vi "读取数据.vi"(8 "error in (no error)":errorcluster, 10 "Slave ID":u8=1, 11 "MB session in":refnum<class "MB_Master.lvclass">) -> (0 "error out":errorcluster, 1 "Registers":u16[](array[numeric]), 2 "读取值":T1 {"累积流量单位" items=["L", "M3", "T", "USG"]; "瞬时流量单位" items=["L/S", "L/M", "L/H", "M3/S", "M3/M", "M3/H", "T/S", "T/M", "T/H", "GPS", "GPM", "GPH"]}, 3 "MB session out":refnum<class "MB_Master.lvclass">)   [LabVIEW 2016, in "MGG-KL-QC流量计.lvlib"]
uses:
  <vilib>/Plasmionique/MB Master/MB_Master/MB_Master.lvclass
  <vilib>/Plasmionique/MB Master/MB Master.lvlib
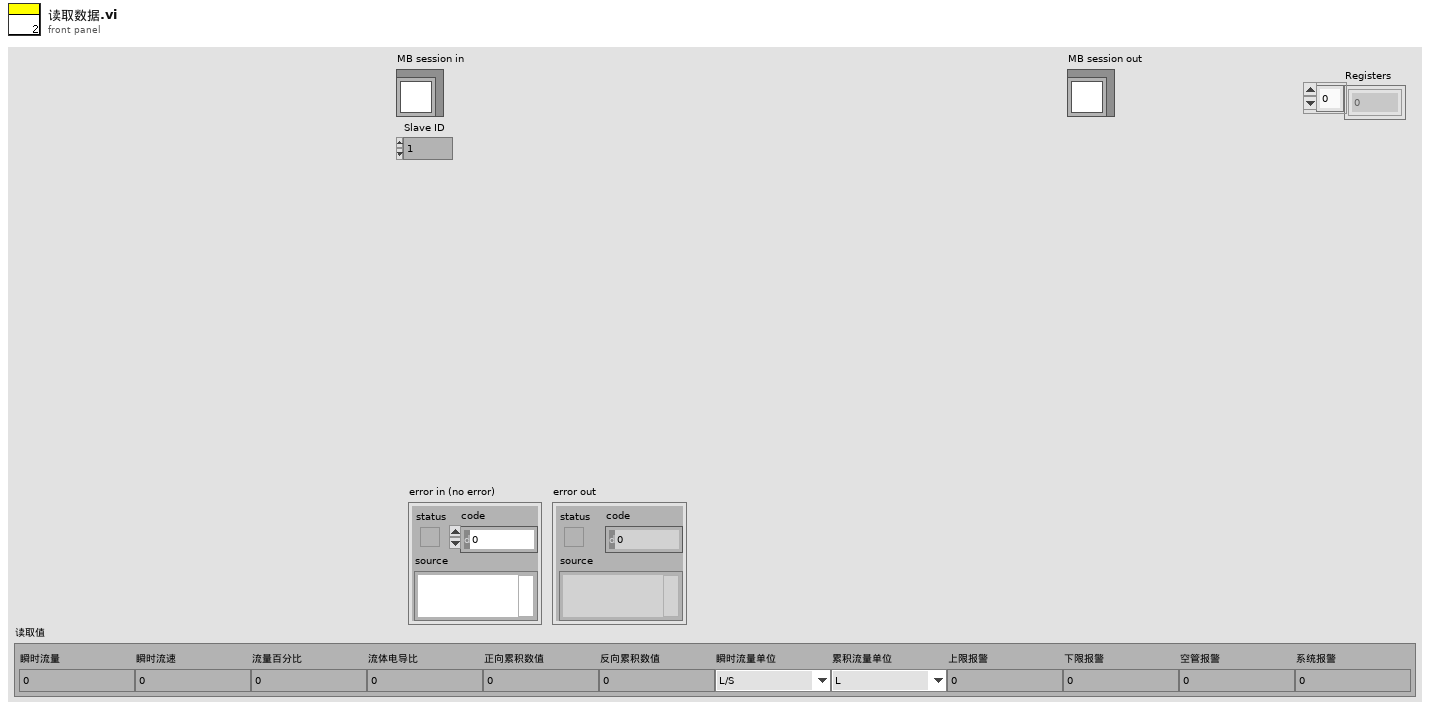
[diagram p1: front panel]
types:
  T1 = typedef "MGG-KL-QC流量计.lvlib/读取值.ctl" = cluster{"瞬时流量":sgl, "瞬时流速":sgl, "流量百分比":sgl, "流体电导比":sgl, "正向累积数值":sgl, "反向累积数值":sgl, "瞬时流量单位":T2, "累积流量单位":T3, "上限报警":u16, "下限报警":u16, "空管报警":u16, "系统报警":u16}
  T2 = typedef "MGG-KL-QC流量计.lvlib/瞬时流量单位.ctl" = u16
  T3 = typedef "MGG-KL-QC流量计.lvlib/累积流量单位.ctl" = u16
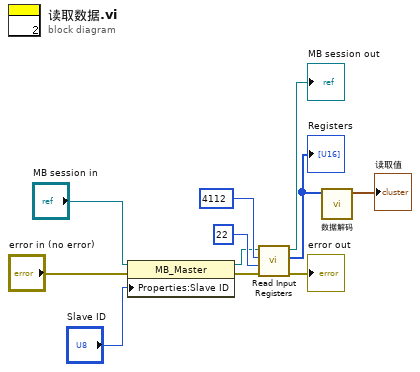
[diagram p0: block diagram]
diagram:
  n1 = property class="MB_Master"(reference="MB session in", error in="error in (no error)", "Properties:Slave ID"="Slave ID") -> (reference out=w4:refnum<class "MB_Master.lvclass">, error out=w2:errorcluster)
  n2 = call <vilib>:"Read Input Registers.vi"("error in (no error)"=w2, "quantity"=u16 22, "starting address"=u16 4112, "MB session in"=w4) -> ("error out"=→"error out":errorcluster, "Registers"=w7:u16[], "MB session out"=→"MB session out":refnum<class "MB_Master.lvclass">)  [unwired: 5 in]
  "Registers" <- w7
  n3 = call "数据解码.vi"("数组"=w7) -> ("读取值"=→"读取值":T1)  [unwired: 10 in]
